vi "test_fit.vi"() -> ()   [LabVIEW 2023]
uses:
  <vilib>/measure/matone.llb/Extract Single Tone Information 1 Chan.vi
  <vilib>/measure/NI_MAPro.lvlib
panel:
  out "detected amplitude":dbl format="%.2p"
  out "detected frequency":dbl format="%.2p"
  out "Waveform Graph":waveform(dbl)(graph)
  in  "N":i32
  in  "Sample rate":dbl
  in  "Phase":dbl
  in  "Amplitude":dbl
  out "Amplitude graph":cluster{dbl[], dbl[]}[](graph)
  out "Phase graph":cluster{dbl[], dbl[]}[](graph)
  out "Actual freq":dbl
  in  "Step":dbl
  in  "Stop freq":dbl
  in  "Start freq":dbl
  in  "Start sweep":bool
  # "Sweep\nparameters"
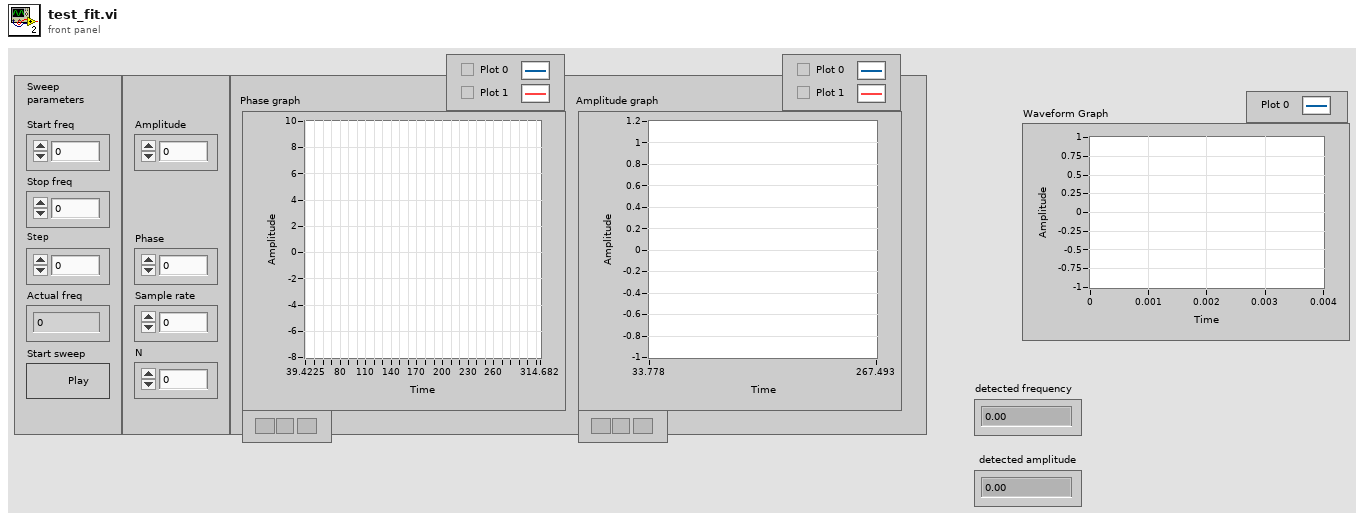
[diagram p1: front panel]
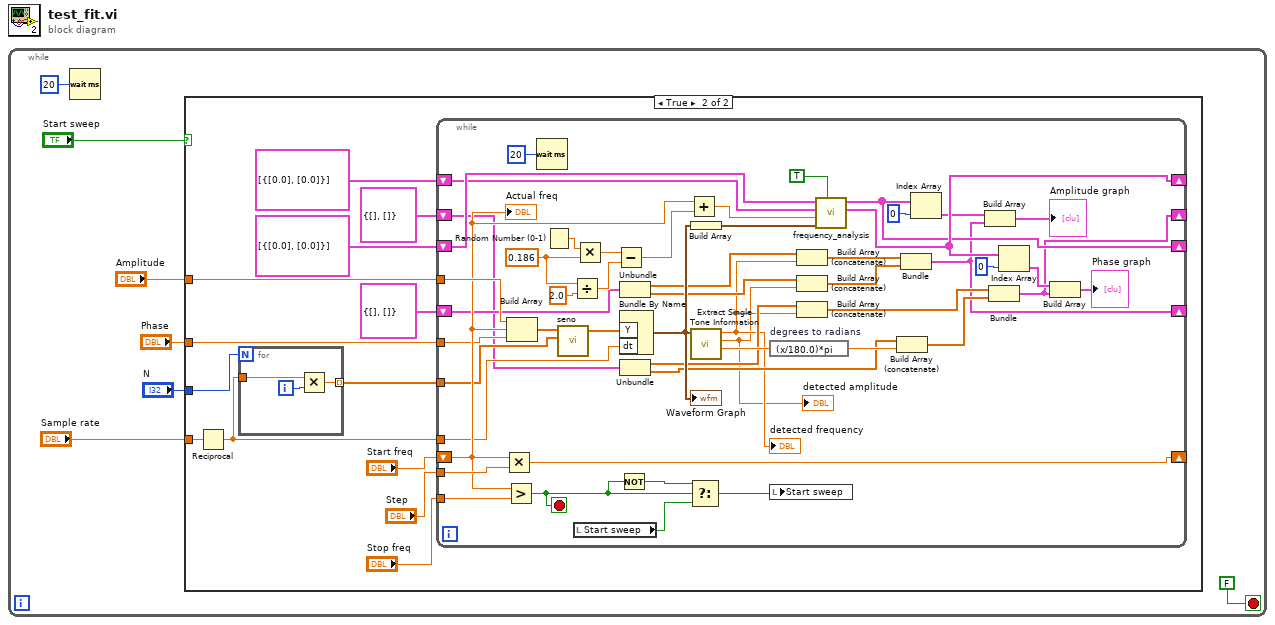
[diagram p0: block diagram]
diagram:
  n1 = while {
    stop <- FALSE stop-if-true
    n2 = Wait (ms)(milliseconds to wait=u32 20) -> ()  [unwired: 1 out]
    n3 = case shown="True" "Start sweep" {
      tunnel: "N" -> [_ w14]
      tunnel: "Sample rate" -> [_ w15]
      tunnel: "Amplitude" -> [_ w17]
      tunnel: "Phase" -> [_ w16]
      frame False {
      }
      frame True {
        n4 = Reciprocal(x=w15) -> (1/x=w12:dbl)
        n5 = for {
          N: w14 -> [_]
          tunnel: w12 -> [w23]
          tunnel: [w21] -> w13 mode=indexing
          i -> [w22]
          n6 = Multiply(x=w23, y=w22) -> (x*y=w21:dbl)
        }
        n7 = while {
          shift-right: [w72] -> _
          shift-left: "Start freq" -> [w61]
          tunnel: "Stop freq" -> [w74]
          tunnel: "Step" -> [w73]
          shift-right: [w46] -> _
          shift-left: cluster{dbl[], dbl[]}[] [{[0.0], [0.0]}] ("XY Amp out") -> [w70]
          shift-right: [w47] -> _
          shift-left: cluster{dbl[], dbl[]}[] [{[0.0], [0.0]}] ("XY Phase out") -> [w69]
          tunnel: w17 -> [w68]
          tunnel: w16 -> [w60]
          tunnel: w12 -> [w51]
          tunnel: w13 -> [w50]
          shift-right: [w33] -> _
          shift-left: cluster{dbl[], dbl[]} {[], []} -> [w30]
          shift-right: [w29] -> _
          shift-left: cluster{dbl[], dbl[]} {[], []} -> [w28]
          stop <- w55 stop-if-true
          w65 = 0.186 ("y")
          n8 = Multiply(x=w61, y=w73) -> (x*y=w72:dbl)
          n9 = Greater?(x=w61, y=w74) -> (0:w55:bool)
          n10 = Build Array(w68, w61, w60) -> (w59:dbl[])
          n11 = Wait (ms)(milliseconds to wait=u32 20) -> ()  [unwired: 1 out]
          n12 = Random Number (0-1)() -> (number: 0 to 1=w67:dbl)
          n13 = call "seno.vi"("X"=w50, "a"=w59) -> ("f(X,a)"=w58:dbl[])  [unwired: 2 in, 2 out]
          n14 = Divide(x=w65, y=2.0) -> (x/y=w63:dbl)
          n15 = local read "Start sweep"() -> (w52:bool)
          n16 = Multiply(x=w67, y=w65) -> (x*y=w66:dbl)
          n17 = Subtract(x=w66, y=w63) -> (x-y=w62:dbl)
          n18 = Not(x=w55) -> (.not. x?=w54:bool)
          n19 = Unbundle(w30) -> (w32:dbl[], w31:dbl[])
          n20 = Bundle By Name("Y"=w58, "dt"=w51) -> (w45:waveform(dbl))  [unwired: 1 in]
          "Waveform Graph" <- w45
          n21 = Unbundle(w28) -> (w27:dbl[], w26:dbl[])
          n22 = Add(x=w61, y=w62) -> (x+y=w44:dbl)
          n23 = Select(t=w54, s=w55, f=w52) -> (s? t:f=w53:bool)
          n24 = Build Array(w45) -> (w57:waveform(dbl)[])
          n25 = call-poly <vilib>:"Extract Single Tone Information.vi"("time signal in"=w45) -> ("detected phase (deg)"=w39:dbl, "detected amplitude"=w24:dbl, "detected frequency"=w25:dbl)  [unwired: 5 in, 3 out]
          "detected frequency" <- w25
          "detected amplitude" <- w24
          n26 = expression code="(x/180.0)*pi" "degrees to radians"(w39) -> (w38:dbl)
          n27 = local write "Start sweep"(w53) -> ()
          n28 = Build Array (concatenate)(w32, w25) -> (w36:dbl[])
          n29 = Build Array (concatenate)(w31, w24) -> (w37:dbl[])
          n30 = Build Array (concatenate)(w27, w25) -> (w34:dbl[])
          n31 = call "frequency_analysis.vi"("Analizza A"=TRUE, "data"=w57, "Fgen freq"=w44, "XY Phase in"=w69, "XY Amp in"=w70) -> ("XY Phase out"=w47:cluster{dbl[], dbl[]}[], "XY Amp out"=w46:cluster{dbl[], dbl[]}[])  [unwired: 5 in]
          n32 = Build Array (concatenate)(w26, w38) -> (w35:dbl[])
          n33 = Bundle(w36, w37) -> (w33:cluster{dbl[], dbl[]})  [unwired: 1 in]
          n34 = Index Array(array=w46, index=0) -> (element=w43:cluster{dbl[], dbl[]})
          n35 = Build Array(w43, w33) -> (→"Amplitude graph":cluster{dbl[], dbl[]}[])
          n36 = Bundle(w34, w35) -> (w29:cluster{dbl[], dbl[]})  [unwired: 1 in]
          n37 = Index Array(array=w47, index=0) -> (element=w41:cluster{dbl[], dbl[]})
          n38 = Build Array(w41, w29) -> (→"Phase graph":cluster{dbl[], dbl[]}[])
          "Actual freq" <- w61
        }
      }
    }
  }
